vi "Write error.vi"(8 "error in (no error)":errorcluster, 10 "error":errorcluster, 11 "Msg_Error.lvclass in":refnum<class "Msg_Error.lvclass">) -> (0 "error out":errorcluster, 3 "Msg_Error.lvclass out":refnum<class "Msg_Error.lvclass">)   [LabVIEW 2012, in "Msg_Error.lvlib" / "Msg_Error.lvclass"]
uses:
  Msg_Error.lvclass
  Msg_Error.lvclass/Msg_Error.ctl
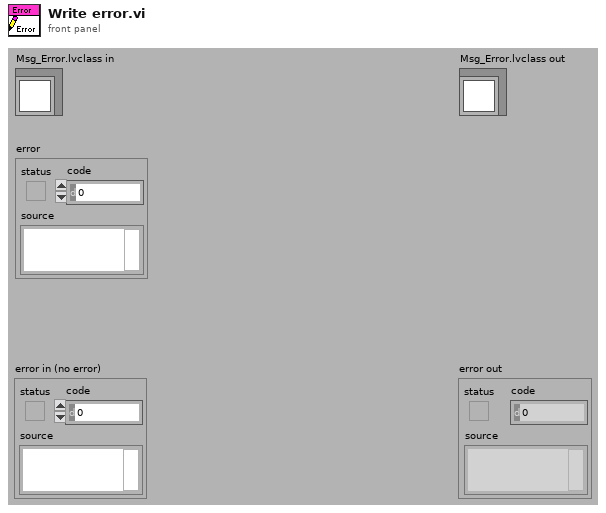
[diagram p1: front panel]
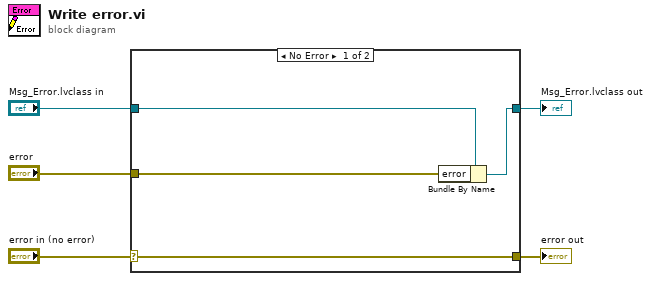
[diagram p0: block diagram]
diagram:
  n1 = case shown="No Error" "error in (no error)" {
    selector: "error in (no error)" -> [w9 w10]
    tunnel: [w9 w10] -> w4
    tunnel: [w7 w11] -> w2
    tunnel: "Msg_Error.lvclass in" -> [w8 w11]
    tunnel: "error" -> [w6 _]
    frame No Error {
      n2 = Bundle By Name(cluster=w8, "error"=w6) -> (w7:refnum<class "Msg_Error.lvclass">)
    }
    frame Error {
    }
  }
  "error out" <- w4
  "Msg_Error.lvclass out" <- w2
